vi "GDSProject_GetFullFolderPath.vi"(1 "Folder Item":refnum<vi>, 5 "error in (no error)":errorcluster) -> (15 "ProjectClassPath":string, 19 "error out":errorcluster)   [LabVIEW 2020]
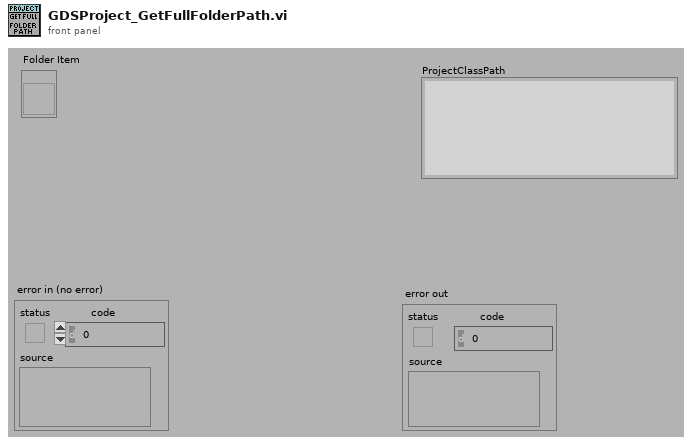
[diagram p1: front panel]
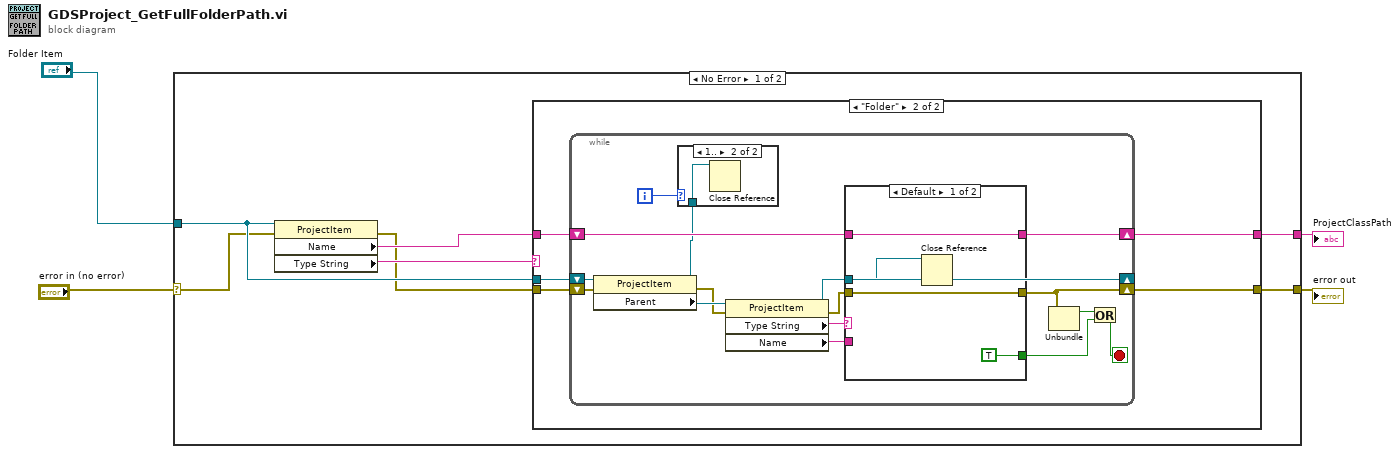
[diagram p0: block diagram]
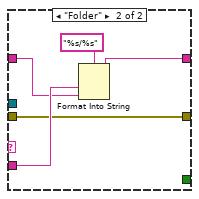
[diagram p3: hidden frame]
diagram:
  n1 = case shown="No Error" "error in (no error)" {
    selector: "error in (no error)" -> [w6 w44]
    tunnel: [w8 w44] -> w3
    tunnel: "Folder Item" -> [w11 _]
    tunnel: [w7 _] -> w1
    frame No Error {
      n2 = property class="ProjectItem"(reference=w11, error in=w6) -> (error out=w5:errorcluster, "Name"=w9:string, "Type String"=w10:string)  [unwired: 1 out]
      n3 = case shown="\"Folder\"" w10 {
        tunnel: w11 -> [_ w17]
        tunnel: w9 -> [_ w16]
        tunnel: w5 -> [w12 w15]
        tunnel: [w12 w14] -> w8
        tunnel: [_ w13] -> w7
        frame Default {
        }
        frame "Folder" {
          n4 = while {
            shift-right: [w18] -> _
            shift-left: w17 -> [w33]
            shift-right: [w21] -> w13
            shift-left: w16 -> [w22]
            shift-right: [w27] -> w14
            shift-left: w15 -> [w28]
            i -> [w32]
            stop <- w24 stop-if-true
            n5 = property class="ProjectItem"(reference=w33, error in=w28) -> (reference out=w19:refnum<vi>, error out=w20:errorcluster, "Parent"=w31:refnum<vi>)
            n6 = case shown="1.." w32 {
              tunnel: w19 -> [_ w43]
              frame 0, Default {
              }
              frame 1.. {
                n7 = Close Reference(reference=w43) -> ()  [unwired: 1 in, 1 out]
              }
            }
            n8 = property class="ProjectItem"(reference=w31, error in=w20) -> (reference out=w18:refnum<vi>, error out=w29:errorcluster, "Type String"=w30:string, "Name"=w23:string)
            n9 = case shown="Default" w30 {
              tunnel: [w37 w38] -> w27
              tunnel: w29 -> [w37 w38]
              tunnel: [TRUE _] -> w25
              tunnel: w23 -> [_ w41]
              tunnel: w22 -> [w35 w40]
              tunnel: [w35 w39] -> w21
              tunnel: w18 -> [w34 _]
              frame Default {
                n10 = Close Reference(reference=w34) -> ()  [unwired: 1 in, 1 out]
              }
              frame "Folder" {
                n11 = Format Into String(format string="%s/%s", w41, w40) -> (resulting string=w39:string)  [unwired: 2 in, 1 out]
              }
            }
            n12 = Unbundle(w27) -> ("status"=w26:bool)  [unwired: 2 out]
            n13 = Or(x=w26, y=w25) -> (x .or. y?=w24:bool)
          }
        }
      }
    }
    frame Error {
    }
  }
  "error out" <- w3
  "ProjectClassPath" <- w1
